vi "Dmadrive.vi"(7 "Operation":T8, 8 "error in (no error)":errorcluster, 10 "Temperature":sgl format="%0.6f", 11 "task":T1={"Task Info"={"Accele Task"=[], "Simulate"=FALSE, "采样率"={"AISampleRate"=10123, "CouplingType"=10000, "Butter"=1000}, "Trig"={"PreTrigCNT"=0, "TriggerMode"=enum."中间触发", "TriggerSource"=enum."软件触发", "ATRTriggerChannel"=enum."通道0", "TriggerDir"=enum."下降沿触发", "TrigLevelVolt"=0.0, "bAvailableTrig"=FALSE}, "clock"={"EN"=FALSE, "clocksource"=enum."内部时钟", "outclocksource"=enum."Trig0"}, "delay(S)"=0.0}, "datain"={"nSegmentCount"=0, "chaneldataSize"=8192, "t0 in"=timestamp(0 s since 1904-01-01), "nsegmentsize"=0, "chanelcouter"=0}, "times"=0.0, "timer"=[], "\nen"=FALSE} {"Task Info"."采样率"."CouplingType" items=["直流耦合", "交流耦合"]}) -> (0 "error out":errorcluster, 1 "data":waveform(dbl)[](array[waveform]), 2 "data?":bool)   [LabVIEW 2009]
uses:
  PCI8532_32.dll
  Ctrls/Enum DAQmx - FGV(V)_Ctrls-某型振动实验台测试系统.ctl
  Ctrls/Acceleration Channel Config_Ctrls-某型振动实验台测试系统.ctl
  Ctrls/Sample Information.ctl
  Ctrls/Trig.ctl
  Ctrls/clock.ctl
  Ctrls/Task Info.ctl
  Ctrls/DATA info.ctl
  Ctrls/task.ctl
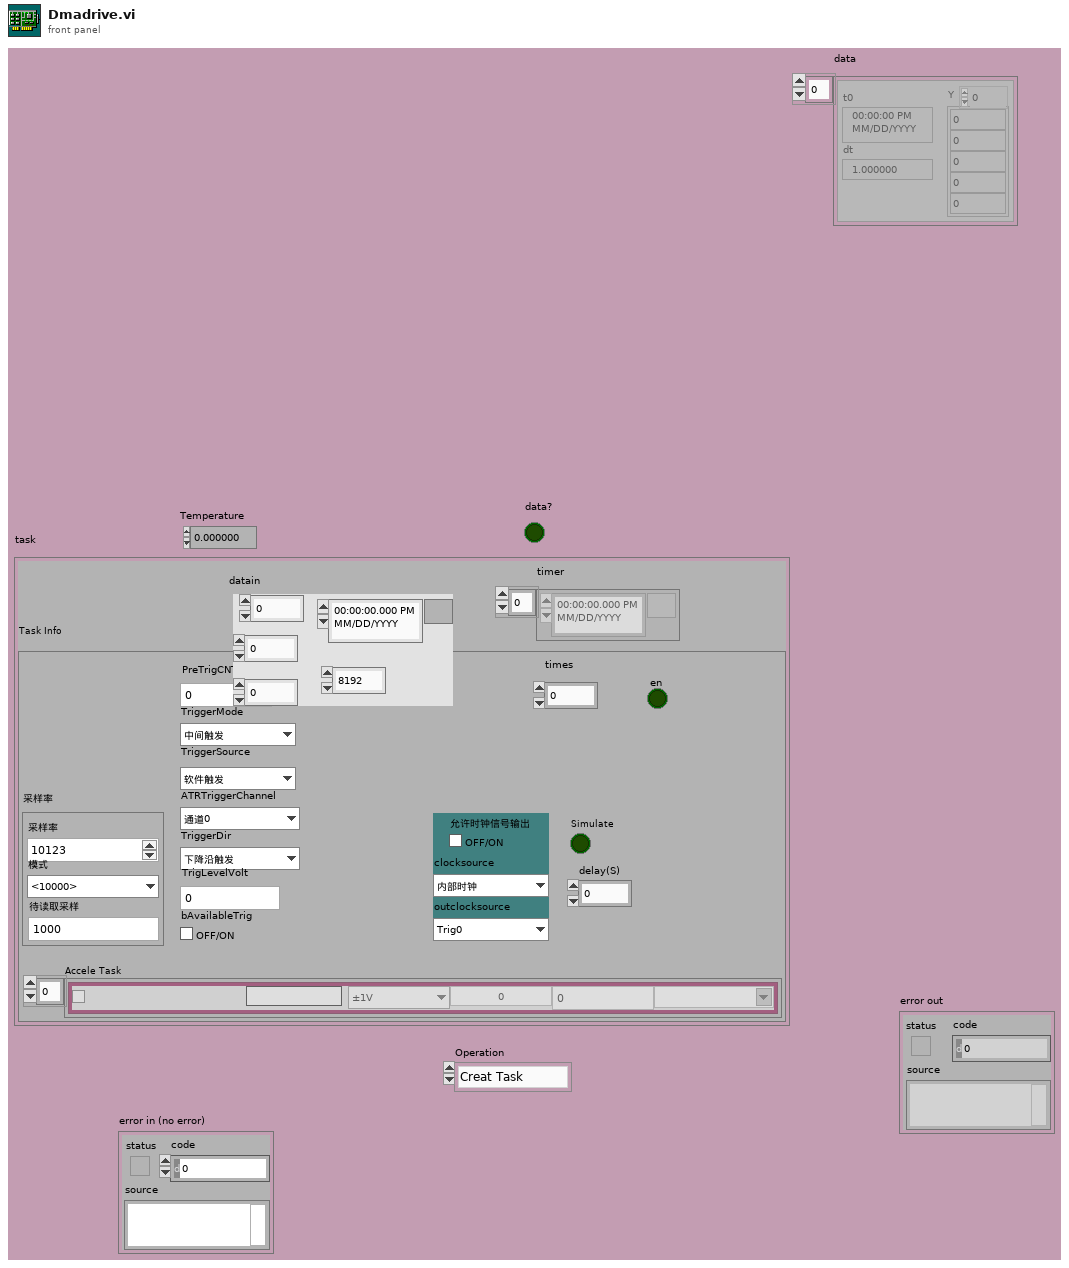
[diagram p1: front panel]
types:
  T1 = typedef "task.ctl" = cluster{"Task Info":T2, "datain":T7, "times":dbl, "timer":timestamp[], "\nen":bool}
  T2 = typedef "Task Info.ctl" = cluster{"Accele Task":T3[], "Simulate":bool, "采样率":T4, "Trig":T5, "clock":T6, "delay(S)":dbl}
  T3 = typedef "Acceleration Channel Config_Ctrls-某型振动实验台测试系统.ctl" = cluster{"Enable":bool, "Name":string, "range":enum16{"±1V", "±5V"}, "SensValue":dbl, "PhysicalName":string, "off":dbl, "Sensunits":string}
  T4 = typedef "Sample Information.ctl" = cluster{"AISampleRate":i32, "CouplingType":i32, "Butter":i32}
  T5 = typedef "Trig.ctl" = cluster{"PreTrigCNT":i32, "TriggerMode":enum16{"中间触发", "后触发", "预触发", "硬件延时触发"}, "TriggerSource":enum16{"软件触发", "DTR信号源", "ATR信号源", "Triger信号触发"}, "ATRTriggerChannel":enum16{"通道0", "通道1", "通道2", "通道3"}, "TriggerDir":enum16{"下降沿触发", "上升沿触发", "上下边没均触发"}, "TrigLevelVolt":sgl, "bAvailableTrig":bool}
  T6 = typedef "clock.ctl" = cluster{"EN":bool, "clocksource":enum16{"内部时钟", "外部时钟"}, "outclocksource":enum16{"Trig0", "Trig1", "Trig2", "Trig3", "Trig4", "Trig5", "Trig6", "Trig7", "PXI_STAR"}}
  T7 = typedef "DATA info.ctl" = cluster{"nSegmentCount":i32, "chaneldataSize":i32, "t0 in":timestamp, "nsegmentsize":i32, "chanelcouter":i32}
  T8 = typedef "Enum DAQmx - FGV(V)_Ctrls-某型振动实验台测试系统.ctl" = enum16{"Creat Task", "Start Task", "Read Data", "Check Task", "Stop Task", "Clear Task"}
  T9 = cluster{"hDevice":i32, "hEvent":i32, "buffer":u16[], "pDMAStatus":i32[]}
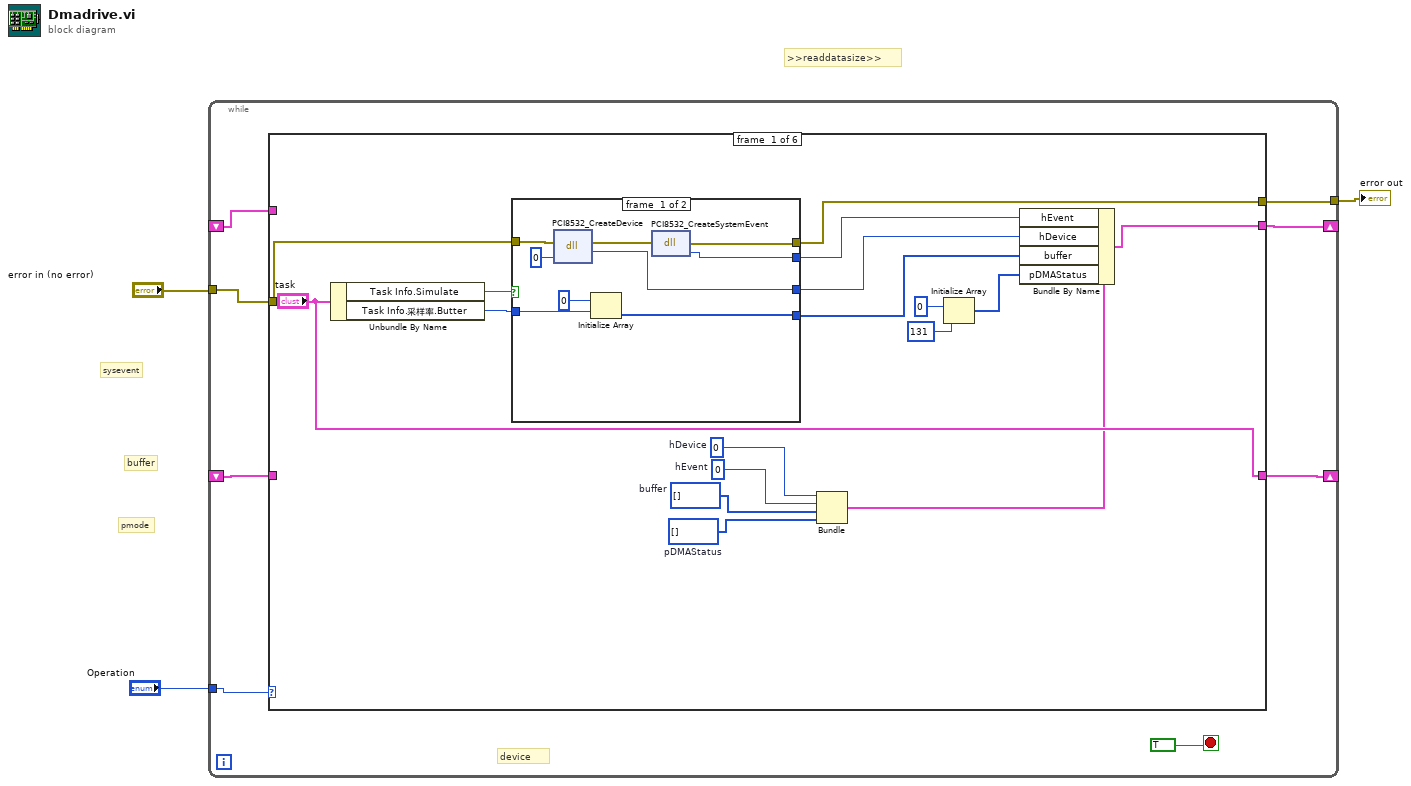
[diagram p0: block diagram]
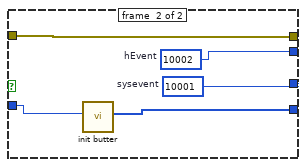
[diagram p2: hidden frame]
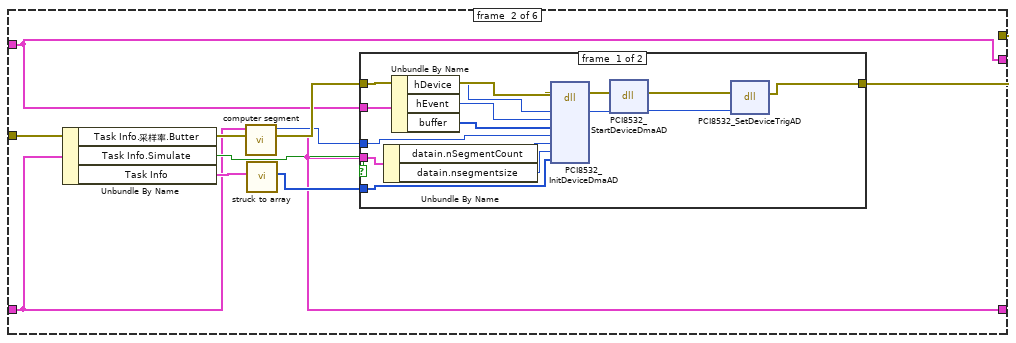
[diagram p3: hidden frame]
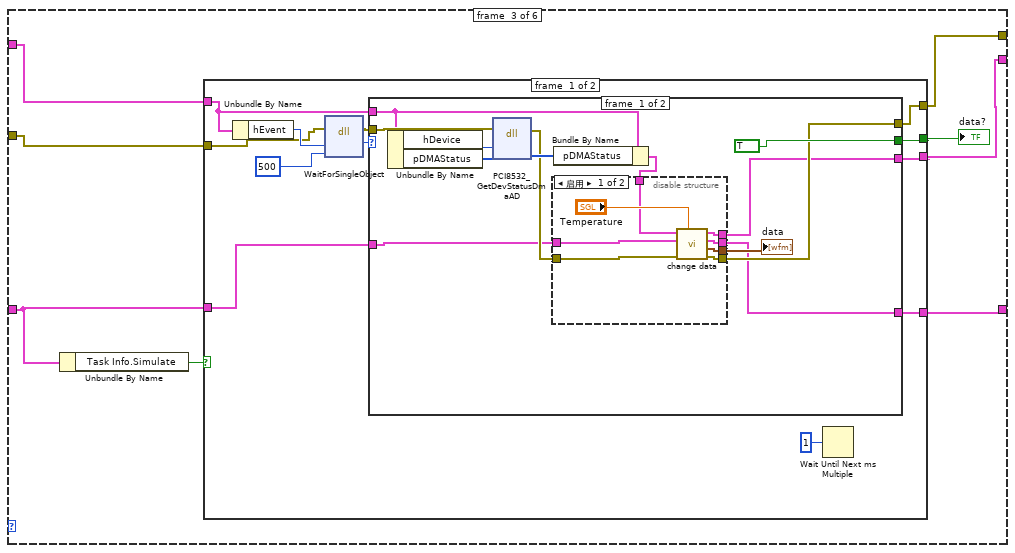
[diagram p5: hidden frame]
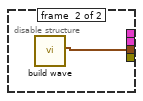
[diagram p6: hidden frame]
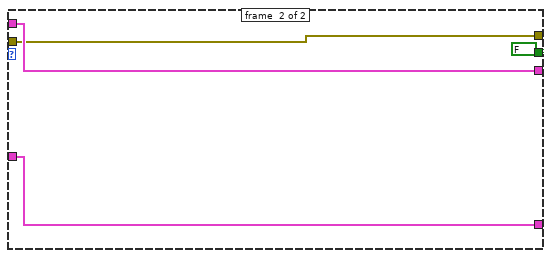
[diagram p7: hidden frame]
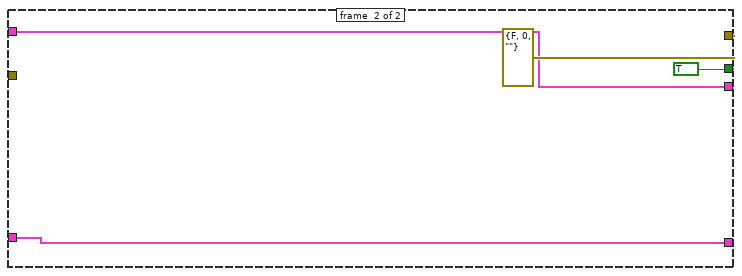
[diagram p8: hidden frame]
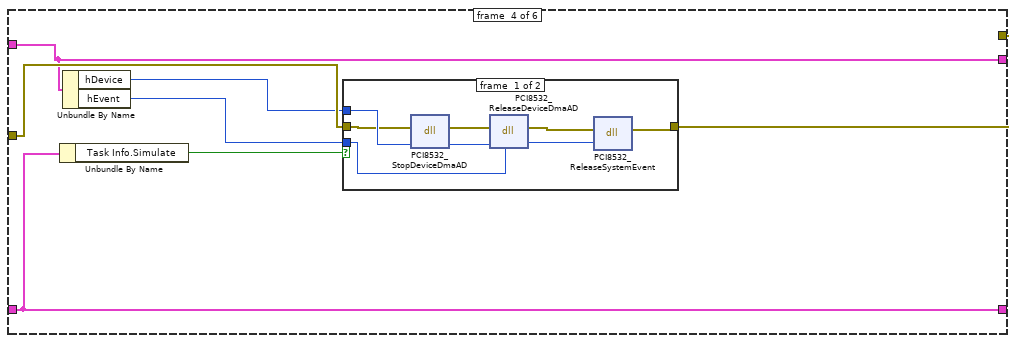
[diagram p9: hidden frame]
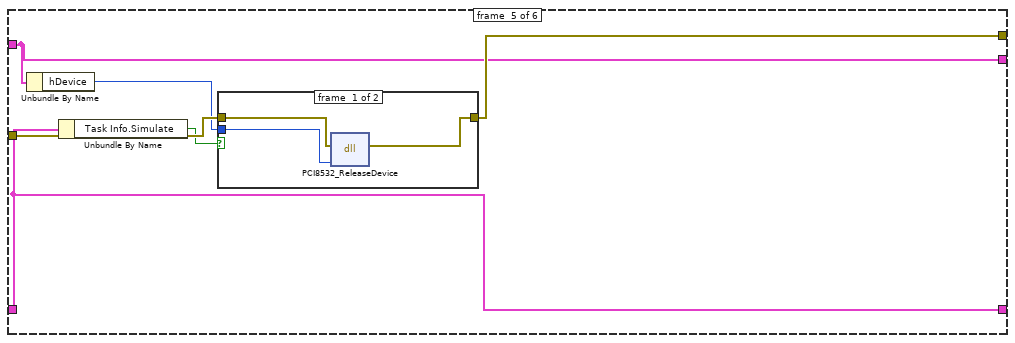
[diagram p11: hidden frame]
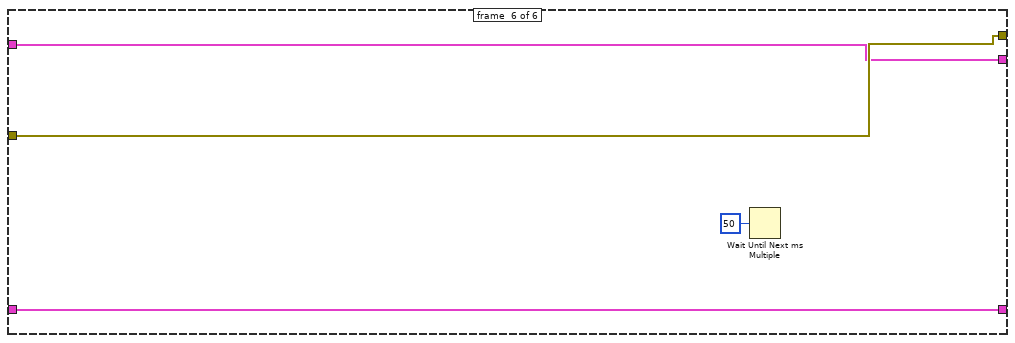
[diagram p13: hidden frame]
diagram:
  # "sysevent"
  # "buffer"
  # ">>readdatasize>>"
  # "pmode"
  n1 = while {
    tunnel: "Operation" -> [w10]
    tunnel: "error in (no error)" -> [w9]
    tunnel: [w8] -> w1
    shift-right: [w6] -> _
    shift-left: _ -> [w7]
    shift-right: [w5] -> _
    shift-left: _ -> [w4]
    stop <- TRUE stop-if-true
    # "device"
    n2 = case shown="\"Read Data\"" w10 {
      tunnel: w9 -> [w26 w52 w69 w125 w139 w147]
      tunnel: [w25 w51 w76 w124 w138 w147] -> w8
      tunnel: w7 -> [_ w45 w75 w123 w137 w145]
      tunnel: ["task" w43 w74 w123 w137 w145] -> w6
      tunnel: [w18 w44 w70 w119 w134 w146] -> w5
      tunnel: w4 -> [_ w44 w71 w119 w134 w146]
      frame #0 {
        w14 = i32[] []  # pDMAStatus
        w21 = u16[] []  # buffer
        w15 = 0  # hDevice
        w16 = 0  # hEvent
        n3 = Unbundle By Name("task") -> ("Task Info.Simulate"=w24:bool, "Task Info.采样率.Butter"=w22:i32)
        n4 = case shown="假" w24 {
          tunnel: [w36 w41] -> w19
          tunnel: [w35 w40] -> w20
          tunnel: w26 -> [w34 w42]
          tunnel: [w32 w42] -> w25
          tunnel: [w31 w38] -> w13
          tunnel: w22 -> [w29 w39]
          frame #0 {
            n5 = dll-call lib="PCI8532_32.dll" fn="PCI8532_CreateDevice" label="CreateDevice"(error in=w34, "DeviceID"=0) -> (error out=w33:errorcluster, "返回类型"=w36:i32)  [unwired: 3 in, 1 out]
            n6 = Initialize Array(u16 0, w29) -> (w31:u16[])
            n7 = dll-call lib="PCI8532_32.dll" fn="PCI8532_CreateSystemEvent" label="CreateSystemEvent"(error in=w33) -> (error out=w32:errorcluster, "hEvent"=w35:i32)  [unwired: 2 in, 1 out]
          }
          frame #1 {
            w40 = 10002  # hEvent
            w41 = 10001  # sysevent
            n8 = call "init butter.vi"("butter"=w39) -> ("init buffer"=w38:u16[])  [unwired: 10 out]
          }
        }
        n9 = Bundle("hDevice"=w15, "hEvent"=w16, "buffer"=w21, "pDMAStatus"=w14) -> (w12:T9)  [unwired: 1 out]
        n10 = Initialize Array ("初始化数组")(0 ("element"), 131 ("dimension size")) -> (w17:i32[])
        n11 = Bundle By Name(cluster=w12, "hEvent"=w20, "hDevice"=w19, "buffer"=w13, "pDMAStatus"=w17) -> (w18:T9)
      }
      frame #1 {
        n12 = Unbundle By Name(w45) -> ("Task Info.采样率.Butter"=w48:i32, "Task Info.Simulate"=w47:bool, "Task Info"=w46:T2)
        n13 = call "computer segment.vi"("Buffer"=w48, "task"=w45) -> ("output cluster"=w43:T1, "nReadsizeword"=w49:i32)  [unwired: 8 out]
        n14 = call "struck to array.vi"("Task Info"=w46) -> ("array"=w50:i32[])  [unwired: 10 out]
        n15 = case shown="假" w47 {
          tunnel: w52 -> [w67 w68]
          tunnel: [w66 w68] -> w51
          tunnel: w50 -> [w63 _]
          tunnel: w49 -> [w60 _]
          tunnel: w44 -> [w59 _]
          tunnel: w43 -> [w56 _]
          frame #0 {
            n16 = Unbundle By Name(w56) -> ("datain.nSegmentCount"=w55:i32, "datain.nsegmentsize"=w54:i32)
            n17 = Unbundle By Name(w59) -> ("hDevice"=w57:i32, "hEvent"=w58:i32, "buffer"=w53:u16[])
            n18 = dll-call lib="PCI8532_32.dll" fn="PCI8532_InitDeviceDmaAD" ("InitDeviceDmaAD")(error in=w67, "hDevice"=w57, "hDmaEvent"=w58, "ADBuffer"=w53, "nReadSizeWords"=w60, "nSegmentCount"=w55, "nSegmentSizeWords"=w54, "pAPara"=w63) -> (error out=w62:errorcluster, "hDevice"=w65:i32)  [unwired: 8 in, 2 out]
            n19 = dll-call lib="PCI8532_32.dll" fn="PCI8532_StartDeviceDmaAD" label="StartDeviceDmaAD"(error in=w62, "hDevice"=w65) -> (error out=w61:errorcluster, "hDevice"=w64:i32)  [unwired: 2 in, 2 out]
            n20 = dll-call lib="PCI8532_32.dll" fn="PCI8532_SetDeviceTrigAD" label="SetDeviceTrigAD"(error in=w61, "hDevice"=w64) -> (error out=w66:errorcluster)  [unwired: 3 in, 2 out]
          }
          frame #1 {
          }
        }
      }
      frame #2 {
        n21 = Unbundle By Name(w75) -> ("Task Info.Simulate"=w72:bool)
        n22 = case shown="假" w72 {
          tunnel: [w82 TRUE] -> w73
          tunnel: [w86 errorcluster {"status"=FALSE, "code"=0, "source"=""} ("error out")] -> w76
          tunnel: w75 -> [w84 w117]
          tunnel: [w83 w117] -> w74
          tunnel: w71 -> [w80 w115]
          tunnel: [w79 w115] -> w70
          tunnel: w69 -> [w78 _]
          frame #0 {
            n23 = Unbundle By Name(w80) -> ("hEvent"=w81:i32)
            n24 = dll-call lib="kernel32" fn="WaitForSingleObject"(error in=w78, "hEvent"=w81, "dwMilliseconds"=500 ("millisecond multiple")) -> (error out=w85:errorcluster, "返回类型"=w77:u32)  [unwired: 4 in, 1 out]
            n25 = case shown="0" w77 {
              tunnel: [w94 w111] -> w86
              tunnel: w84 -> [w90 w114]
              tunnel: [w89 w114] -> w83
              tunnel: w85 -> [w101 w111]
              tunnel: [TRUE FALSE] -> w82
              tunnel: w80 -> [w96 w112]
              tunnel: [w92 w112] -> w79
              frame #0 {
                n26 = Unbundle By Name(w96) -> ("hDevice"=w99:i32, "pDMAStatus"=w98:i32[])
                n27 = dll-call lib="PCI8532_32.dll" fn="PCI8532_GetDevStatusDmaAD" ("GetDevStatusDmaAD")(error in=w101, "hDevice"=w99, "pDMAStatus"=w98) -> (error out=w93:errorcluster, "pDMAStatus"=w97:i32[])  [unwired: 2 in, 3 out]
                n28 = Bundle By Name(cluster=w96, "pDMAStatus"=w97) -> (w91:T9)
                n29 = disable-structure shown="启用" {
                  disable-tunnel: [w109 w110] -> w95
                  disable-tunnel: [w107 _] -> w94
                  disable-tunnel: w93 -> [w106 _]
                  disable-tunnel: [w105 _] -> w92
                  disable-tunnel: w91 -> [w104 _]
                  disable-tunnel: w90 -> [w103 _]
                  disable-tunnel: [w102 _] -> w89
                  frame #0 {
                    n30 = call "change data.vi"("register in"=w104, "task in"=w103, "error in"=w106, "Temperature"="Temperature") -> ("register out"=w105:T9, "task out"=w102:T1, "data"=w109:waveform(dbl)[], "error out"=w107:errorcluster)  [unwired: 1 in, 2 out]
                  }
                  frame #1 {
                    n31 = call "build wave.vi"() -> ("数组"=w110:waveform(dbl)[])  [unwired: 11 out]
                  }
                }
                "data" <- w95
              }
              frame #1 {
              }
            }
            n32 = Wait Until Next ms Multiple(millisecond multiple=u32 1) -> ()  [unwired: 1 out]
          }
          frame #1 {
          }
        }
        "data?" <- w73
      }
      frame #3 {
        n33 = Unbundle By Name(w123) -> ("Task Info.Simulate"=w122:bool)
        n34 = Unbundle By Name(w119) -> ("hDevice"=w121:i32, "hEvent"=w120:i32)
        n35 = case shown="假" w122 {
          tunnel: w121 -> [w131 _]
          tunnel: w125 -> [w130 w133]
          tunnel: [w127 w133] -> w124
          tunnel: w120 -> [w126 _]
          frame #0 {
            n36 = dll-call lib="PCI8532_32.dll" fn="PCI8532_StopDeviceDmaAD" ("StopDeviceDmaAD")(error in=w130, "hDevice"=w131) -> (error out=w129:errorcluster, "hDevice"=w132:i32)  [unwired: 2 in, 2 out]
            n37 = dll-call lib="PCI8532_32.dll" fn="PCI8532_ReleaseDeviceDmaAD" ("ReleaseDeviceDmaAD")(error in=w129, "hDevice"=w132) -> (error out=w128:errorcluster)  [unwired: 3 in, 2 out]
            n38 = dll-call lib="PCI8532_32.dll" fn="PCI8532_ReleaseSystemEvent" ("ReleaseSystemEvent")(error in=w128, "hEvent"=w126) -> (error out=w127:errorcluster)  [unwired: 3 in, 2 out]
          }
          frame #1 {
          }
        }
      }
      frame #4 {
        n39 = Unbundle By Name(w134) -> ("hDevice"=w135:i32)
        n40 = Unbundle By Name(w137) -> ("Task Info.Simulate"=w136:bool)
        n41 = case shown="假" w136 {
          tunnel: w135 -> [w142 _]
          tunnel: w139 -> [w141 w143]
          tunnel: [w140 w143] -> w138
          frame #0 {
            n42 = dll-call lib="PCI8532_32.dll" fn="PCI8532_ReleaseDevice" label="ReleaseDevice"(error in=w141, "hDevice"=w142) -> (error out=w140:errorcluster)  [unwired: 3 in, 2 out]
          }
          frame #1 {
          }
        }
      }
      frame #5 {
        n43 = Wait Until Next ms Multiple(millisecond multiple=u32 50 ("毫秒倍数")) -> ()  [unwired: 1 out]
      }
    }
  }
  "error out" <- w1
